vi "Open Sensors V.3.0.vi"   [LabVIEW 2017]
uses:
  <vilib>/Rock Robotics/SystemInterfaces/DIO/FPGA_DIOChannel.ctl
  <vilib>/Rock Robotics/SystemInterfaces/AI/FPGA_AIChannel.ctl
  <vilib>/Rock Robotics/SystemInterfaces/spilib/spi_bus.ctl
  <vilib>/Rock Robotics/WPI/Gyro/WPI_GyroXRS450_SPI_Open.vi
types:
  T1 = typedef "spi_bus.ctl" = enum16{"SPI On-Board, CS0", "SPI On-Board, CS1", "SPI On-Board, CS2", "SPI On-Board, CS3", "SPI MXP", "Invalid"}
  T2 = typedef "FPGA_AIChannel.ctl" = enum8{"AI 0", "AI 1", "AI 2", "AI 3", "AI MXP 0", "AI MXP 1", "AI MXP 2", "AI MXP 3", "Invalid"}
  T3 = typedef "FPGA_DIOChannel.ctl" = enum8{"DIO 0", "DIO 1", "DIO 2", "DIO 3", "DIO 4", "DIO 5", "DIO 6", "DIO 7", "DIO 8", "DIO 9", "DIO MXP 0", "DIO MXP 1", "DIO MXP 2", "DIO MXP 3", "DIO MXP 4", "DIO MXP 5", "DIO MXP 6", "DIO MXP 7", "DIO MXP 8", "DIO MXP 9", "DIO MXP 10", "DIO MXP 11", "DIO MXP 12", "DIO MXP 13", "DIO MXP 14", "DIO MXP 15", "SPI Port CS1", "SPI Port CS2", "SPI Port CS3", "SPI Port MISO", "SPI Port MOSI", "Invalid"}
  T4 = typedef "WPI_GyroDevRef.ctl" = cluster{"DevStatus":errorcluster, "Analog Channel":T2, "Gain (VoltsPerDegree/Second)":dbl, "Gyro Type":enum16{"Analog", "XRS450"}, "Handle":i32, "SPI Bus":T1, "Device Found":bool, "Sample Rate":dbl, "Calibrate On Open":bool, "Offset":dbl}
  T5 = typedef "WPI_DigitalInputDevRef.ctl" = cluster{"DevStatus":errorcluster, "DIO Channel":T3}
  T6 = typedef "WPI_PotentiometerDevRef.ctl" = cluster{"DevStatus":errorcluster, "Analog Channel":T2, "Invert Output":bool}
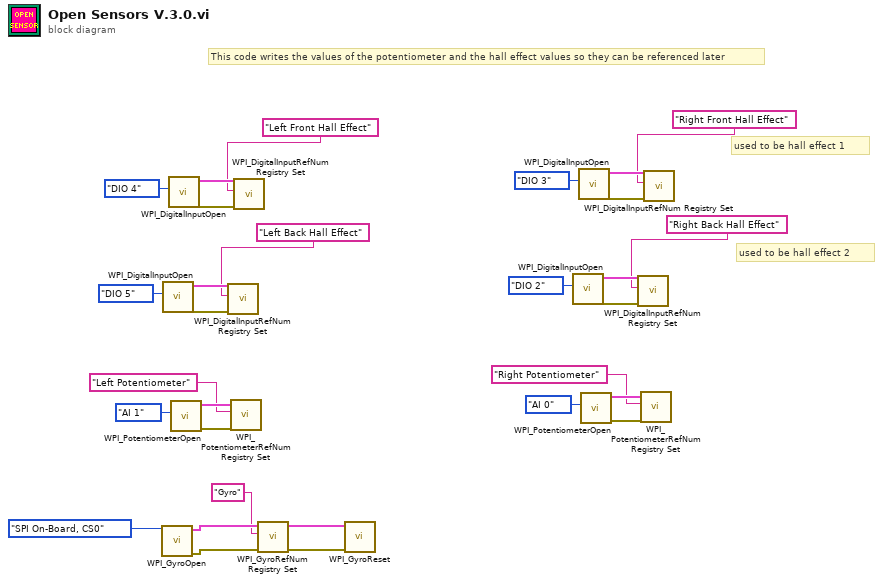
[diagram p0: block diagram]
diagram:
  # "This code writes the values of the potentiometer and the hall effect values so they can be referenced later"
  # "used to be hall effect 1"
  # "used to be hall effect 2"
  n1 = call-poly <vilib>:"WPI_GyroOpen.vi"("SPI Bus"=spi_bus."SPI On-Board, CS0") -> ("error out"=w5:errorcluster, "GyroDevRef"=w6:T4)  [unwired: 8 in, 1 out]
  n2 = call <vilib>:"WPI_DigitalInputOpen.vi"("DIO Channel"=FPGA_DIOChannel."DIO 5") -> ("error out"=w16:errorcluster, "DigitalInputDevRef"=w17:T5)  [unwired: 9 in]
  n3 = call <vilib>:"WPI_DigitalInputOpen.vi"("DIO Channel"=FPGA_DIOChannel."DIO 4") -> ("error out"=w12:errorcluster, "DigitalInputDevRef"=w13:T5)  [unwired: 9 in]
  n4 = call <vilib>:"WPI_PotentiometerOpen.vi"("Analog Channel"=FPGA_AIChannel."AI 1") -> ("error out"=w10:errorcluster, "PotDevRef"=w9:T6)  [unwired: 9 in]
  n5 = call <vilib>:"WPI_DigitalInputRefNum Registry Set.vi"("error in (no error)"=w16, "refnum name"="Left Back Hall Effect", "DigitalInputDevRef"=w17) -> ()  [unwired: 7 in, 2 out]
  n6 = call <vilib>:"WPI_PotentiometerRefNum Registry Set.vi"("error in (no error)"=w10, "refnum name"="Left Potentiometer", "PotDevRef"=w9) -> ()  [unwired: 7 in, 2 out]
  n7 = call <vilib>:"WPI_DigitalInputRefNum Registry Set.vi"("error in (no error)"=w12, "refnum name"="Left Front Hall Effect", "DigitalInputDevRef"=w13) -> ()  [unwired: 7 in, 2 out]
  n8 = call <vilib>:"WPI_GyroRefNum Registry Set.vi"("error in (no error)"=w5, "refnum name"="Gyro", "GyroDevRef"=w6) -> ("error out"=w3:errorcluster, "GyroDevRef"=w4:T4)  [unwired: 7 in]
  n9 = call <vilib>:"WPI_GyroReset.vi"("error in"=w3, "GyroDevRef"=w4) -> ()  [unwired: 8 in, 2 out]
  n10 = call <vilib>:"WPI_DigitalInputOpen.vi"("DIO Channel"=FPGA_DIOChannel."DIO 2") -> ("error out"=w28:errorcluster, "DigitalInputDevRef"=w29:T5)  [unwired: 9 in]
  n11 = call <vilib>:"WPI_DigitalInputOpen.vi"("DIO Channel"=FPGA_DIOChannel."DIO 3") -> ("error out"=w24:errorcluster, "DigitalInputDevRef"=w25:T5)  [unwired: 9 in]
  n12 = call <vilib>:"WPI_PotentiometerOpen.vi"("Analog Channel"=FPGA_AIChannel."AI 0") -> ("error out"=w22:errorcluster, "PotDevRef"=w21:T6)  [unwired: 9 in]
  n13 = call <vilib>:"WPI_DigitalInputRefNum Registry Set.vi"("error in (no error)"=w28, "refnum name"="Right Back Hall Effect", "DigitalInputDevRef"=w29) -> ()  [unwired: 7 in, 2 out]
  n14 = call <vilib>:"WPI_PotentiometerRefNum Registry Set.vi"("error in (no error)"=w22, "refnum name"="Right Potentiometer", "PotDevRef"=w21) -> ()  [unwired: 7 in, 2 out]
  n15 = call <vilib>:"WPI_DigitalInputRefNum Registry Set.vi"("error in (no error)"=w24, "refnum name"="Right Front Hall Effect", "DigitalInputDevRef"=w25) -> ()  [unwired: 7 in, 2 out]
